vi "xcorr_test.vi"() -> ()   [LabVIEW 2012]
uses:
  <vilib>/gmath/NI_Gmath.lvlib
panel:
  out "Array 3":dbl[](array[numeric])
  out "Array 2":dbl[](array[numeric])
  out "Array":dbl[][](array[numeric])
  in  "data":dbl[][](array[numeric])
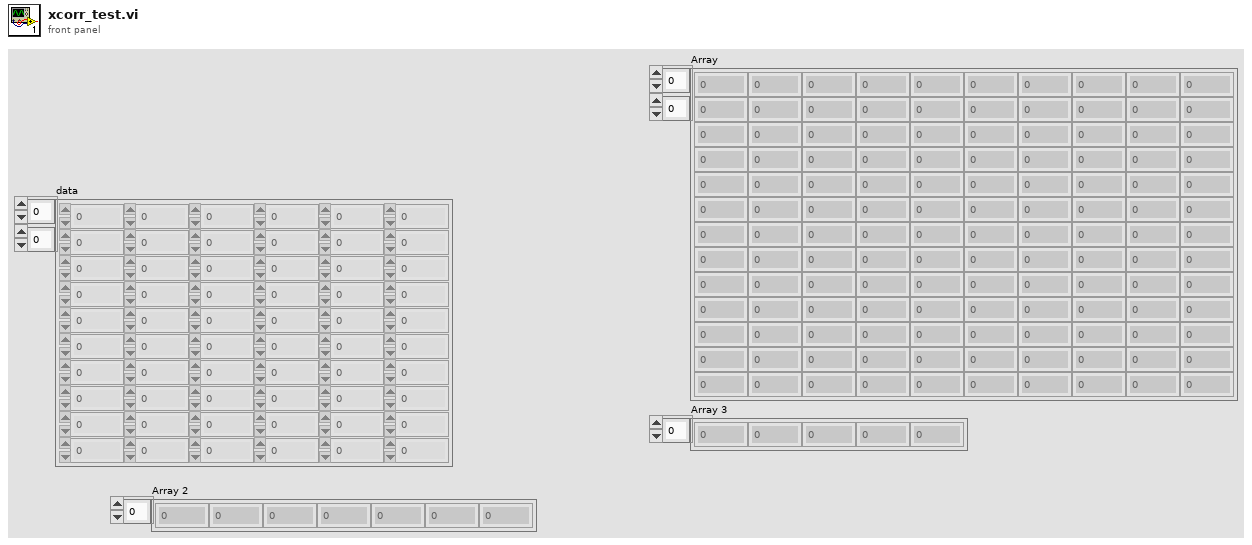
[diagram p1: front panel]
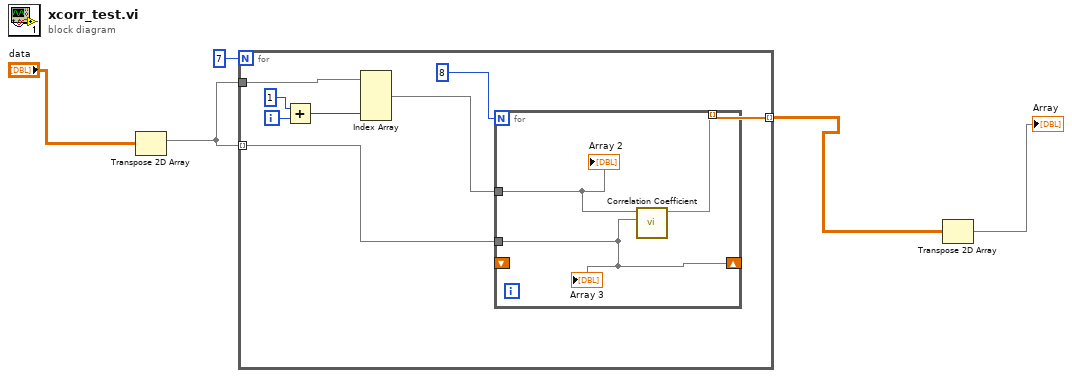
[diagram p0: block diagram]
diagram:
  n1 = Transpose 2D Array(2D array="data") -> (transposed array=w3:dbl[][])
  n2 = for {
    N: 7 -> [_]
    tunnel: [w13] -> w2 mode=indexing
    tunnel: w3 -> [w6] mode=indexing
    tunnel: w3 -> [w9]
    i -> [w12]
    n3 = Add(x=1, y=w12) -> (x+y=w10:i32)
    n4 = Index Array(array=w9, index (row) #1=w10) -> (element #1=w8:dbl[])  [unwired: 3 in, 1 out]
    n5 = for {
      N: 8 -> [_]
      tunnel: [w16] -> w13 mode=indexing
      tunnel: w8 -> [w15]
      tunnel: w6 -> [w14]
      shift-right: [w14] -> _
      shift-left: _ -> [_]
      n6 = call <vilib>:"Correlation Coefficient.vi"("Y"=w14, "X"=w15) -> ("correlation coefficient r"=w16:dbl)  [unwired: 8 in, 1 out]
      "Array 2" <- w15
      "Array 3" <- w14
    }
  }
  n7 = Transpose 2D Array(2D array=w2) -> (transposed array=→"Array":dbl[][])
